vi "Get events counter.vi"(8 "error in (no error)":errorcluster caption="entrée d'erreur (pas d'erreur)", 11 "DAQmxTaskContainer_general en entrée":refnum<class "DAQmxTaksContainer_General.lvclass">) -> (0 "error out":errorcluster caption="sortie d'erreur", 2 "events counter":refnum<user-event>[](array[refnum]), 3 "DAQmxTaskContainer_general en sortie":refnum<class "DAQmxTaksContainer_General.lvclass">)   [LabVIEW 2015]
uses:
  DAQmxTaksContainer_General.lvclass
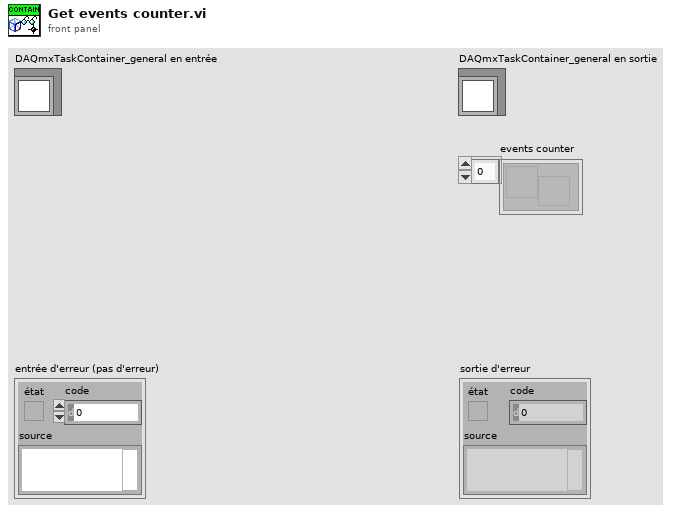
[diagram p1: front panel]
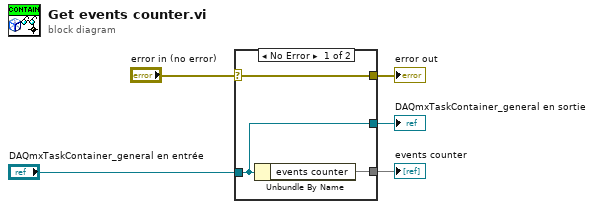
[diagram p0: block diagram]
diagram:
  n1 = case shown="No Error" "error in (no error)" {
    selector: "error in (no error)" -> [w8 w9]
    tunnel: [w8 w9] -> w4
    tunnel: [w7 w10] -> w2
    tunnel: "DAQmxTaskContainer_general en entrée" -> [w7 w10]
    tunnel: [w6 _] -> w1
    frame No Error {
      n2 = Unbundle By Name(w7) -> ("events counter"=w6)
    }
    frame Error {
    }
  }
  "error out" <- w4
  "DAQmxTaskContainer_general en sortie" <- w2
  "events counter" <- w1
